vi "Pixelfly AE.vi"(7 "Action":enum16{"READ", "WRITE"}(ring), 10 "Gate Delay Ref In":refnum<vi>) -> (2 "Gate Delay Ref Out":refnum<vi>)   [LabVIEW 2014]
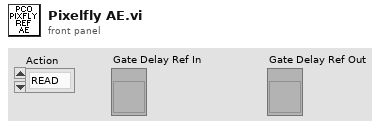
[diagram p1: front panel]
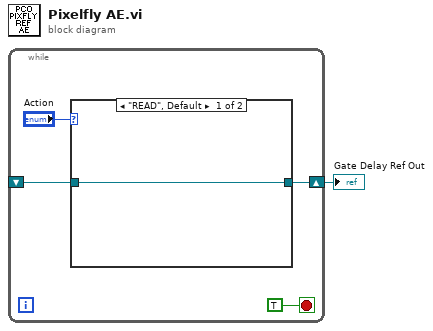
[diagram p0: block diagram]
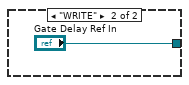
[diagram p2: hidden frame]
diagram:
  n1 = while {
    shift-right: [w3] -> w1
    shift-left: _ -> [w2]
    stop <- TRUE stop-if-true
    n2 = case shown="\"READ\", Default" "Action" {
      tunnel: [w6 "Gate Delay Ref In"] -> w3
      tunnel: w2 -> [w6 _]
      frame "READ", Default {
      }
      frame "WRITE" {
      }
    }
  }
  "Gate Delay Ref Out" <- w1
